vi "note value scripting.vi"   [LabVIEW 2020]
uses:
  midi-file/Note Value.ctl
  <vilib>/Utility/traverseref.llb/TRef TravTarget.ctl
  midi-file/midi-file.lvclass
types:
  T1 = typedef "TRef TravTarget.ctl" = enum16{"FP", "BD", "Other"}
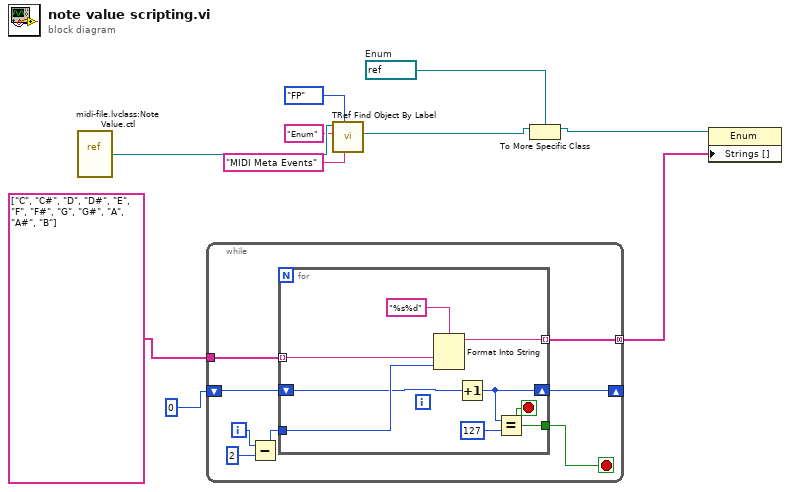
[diagram p0: block diagram]
diagram:
  w4 = refnum<vi> refnum  # Enum
  n1 = vi-ref "midi-file.lvclass:Note Value.ctl"() -> (w9:refnum<vi>)
  n2 = while {
    tunnel: string[] ["C", "C#", "D", "D#", "E", "F", "F#", "G", "G#", "A", "A#", "B"] -> [w18]
    tunnel: [w13] -> w2 mode=concatenating
    shift-right: [w11] -> _
    shift-left: 0 ("y") -> [w12]
    i -> [w16]
    stop <- w17 stop-if-true
    n3 = Subtract(x=w16, y=2) -> (x-y=w14:i32)
    n4 = for {
      tunnel: w14 -> [w26]
      tunnel: w18 -> [w25] mode=indexing
      tunnel: [w19] -> w17
      tunnel: [w23] -> w13 mode=indexing
      shift-right: [w21] -> w11
      shift-left: w12 -> [w20]
      stop <- w19 stop-if-true
      n5 = Format Into String(format string="%s%d", w25, w26) -> (resulting string=w23:string)  [unwired: 2 in, 1 out]
      n6 = Increment(x=w20) -> (x+1=w21:i32)
      n7 = Equal?(x=w21, y=127) -> (x = y?=w19:bool)
    }
  }
  n8 = call <vilib>:"TRef Find Object By Label.vi"("Label"="MIDI Meta Events", "Traverse Target"=TRef_TravTarget."FP", "Class Name"="Enum", "VI Ref"=w9) -> ("Found Obj Ref"=w5:refnum<vi>)  [unwired: 4 in, 3 out]
  n9 = To More Specific Class(target class=w4, reference=w5) -> (specific class reference=w3:refnum<vi>)  [unwired: 1 in, 1 out]
  n10 = property class="Enum"(reference=w3, "Strings []"=w2) -> ()  [unwired: 1 in, 2 out]
